vi "Rand W.vi"(2 "Weight gain":dbl, 4 "post":i32[][](array[numeric]), 5 "Occupied":i32[](array[numeric])) -> (0 "W Array":dbl[](array[numeric]))   [LabVIEW 2013]
uses:
  <vilib>/gmath/statdist.llb/Normal Random.vi
  <vilib>/gmath/NI_Gmath.lvlib
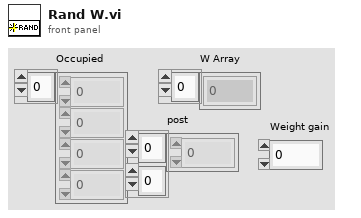
[diagram p1: front panel]
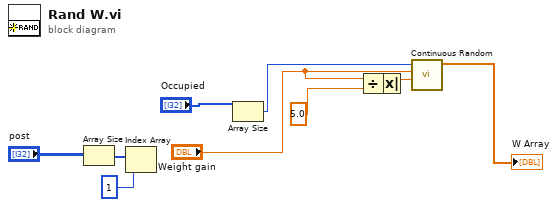
[diagram p0: block diagram]
diagram:
  n1 = Array Size(array="post") -> (size(s)=w9:i32[])
  n2 = Index Array(array=w9, index=1) -> ()  [unwired: 1 out]
  n3 = Array Size(array="Occupied") -> (size(s)=w5:i32)
  n4 = Divide(x="Weight gain", y=5.0) -> (x/y=w3:dbl)
  n5 = Absolute Value(x=w3) -> (abs(x)=w1:dbl)
  n6 = call-poly <vilib>:"Continuous Random.vi"("std"=w1, "mean"="Weight gain", "samples"=w5) -> ("normal random data"=→"W Array":dbl[])  [unwired: 7 in, 1 out]
